vi "CSGaussmeter.setAuto.vi"(0 "i ref in":refnum<vi>, 7 "Auto":bool, 11 "error in (no error)":errorcluster) -> (4 "i ref out":refnum<vi>, 15 "error out":errorcluster)   [LabVIEW 2014, in "CSGaussmeter.lvlib"]
doc: "This VI sets the Auto Range ON or OFF. \n\nDurch das VI Auto_Range kann die automatische Messbereichswahl eingeschaltet werden."
uses:
  CSGaussmeter.lvlib
  CSCore/CSObj/CSObj.lvlib
  CSlibraries/UtilityLib/UtilityLib.lvlib
  CSinstr.lib/FH_55/FH 55.lvlib
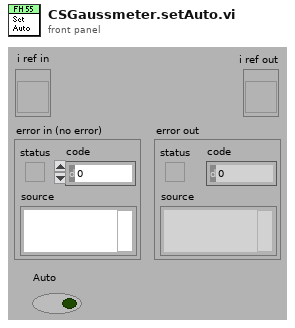
[diagram p1: front panel]
types:
  T1 = typedef "CSGaussmeter.lvlib/CSGaussmeter.i attribute.ctl" = cluster{"Name":string, "VISA Resource Name":refnum<visa-resource-name>, "actValues":cluster{" Limit":bool, "Unit ":T2, "Temp_Unit":T3, "Max":T4, " Filter":bool, " Peak":bool, " Auto_Range":bool, "Range":T5, " Rel":bool, " CTemp":bool, " CField":bool, "AC_DC ":bool, "Set_lower":cluster{"Numeric":dbl, "Cancel Button":bool, "Unit":T6}, "Set_upper":cluster{"Numeric":dbl, "Cancel Button":bool, "Unit":T6}, "Set_Rel":cluster{"Numeric":dbl, "Cancel Button":bool, "Unit":T6}, "Zero":bool, " Local":bool, "Reset":bool, " Init":bool}, "FH 55 Gauss-/Teslameter":T7, "MAX_Value":T8, "MIN_Value":T8, "Rel_Value":T8, "Array ":string[], "LIMU":dbl, " LIML":dbl, "Messwerte 2":string, "Messwerte ":cluster{"Numeric":i32, "OK Button":bool}, "serviceID":cluster{"Current ID":i32, "Unit ID":i32, "Temp ID":i32, "Name ID \n":i32, "Visa ID ":i32}, "setValues ":cluster{" Limit":bool, "Unit ":T2, "Temp_Unit":T3, "Max":T4, " Filter":bool, " Peak":bool, " Auto_Range":bool, "Range":T5, " Rel":bool, " CTemp":bool, " CField":bool, "AC_DC ":bool, "Set_lower":cluster{"Numeric":dbl, "Cancel Button":bool, "Unit":T6}, "Set_upper":cluster{"Numeric":dbl, "Cancel Button":bool, "Unit":T6}, "Set_Rel":cluster{"Numeric":dbl, "Cancel Button":bool, "Unit":T6}, "Zero":bool, " Local":bool, "Reset":bool, " Init":bool}}
  T2 = typedef "FH 55.lvlib/Unit.ctl" = enum16{"T", "G", "A/m"}
  T3 = typedef "FH 55.lvlib/Temp_Unit.ctl" = enum16{"Temp off", "Celsius", "Fahrenheit"}
  T4 = typedef "FH 55.lvlib/Max.ctl" = enum16{"MAX off", "Show MAX", "MAX/MIN"}
  T5 = typedef "FH 55.lvlib/Range.ctl" = enum16{"1", "2", "3", "4", "5", "6", "7"}
  T6 = typedef "FH 55.lvlib/Unit2.ctl" = enum16{"mT", "G", "kA/m"}
  T7 = typedef "FH 55.lvlib/Display.ctl" = cluster{"current value":string, "Limit":string, "Remote":string, "function ":string, "Cluster":cluster{"AC/DC":string, "Auto":string, "Filter":string, "Range":string, "Rel":string, "Peak":string}}
  T8 = typedef "FH 55.lvlib/Value_String.ctl" = cluster{"Numeric":dbl, "String":string}
  T9 = cluster{"VISA Resource Name":refnum<visa-resource-name>}
  T10 = typedef "FH 55.lvlib/VisaCluster.ctl" = cluster{"VISA Resource Name":refnum<visa-resource-name>}
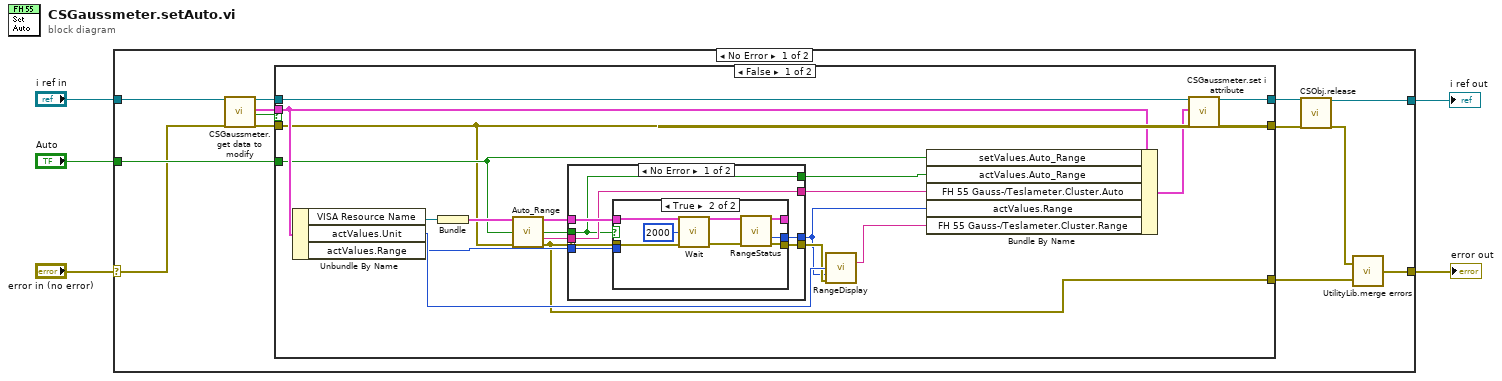
[diagram p0: block diagram]
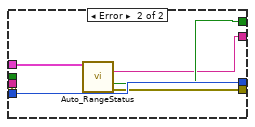
[diagram p3: hidden frame]
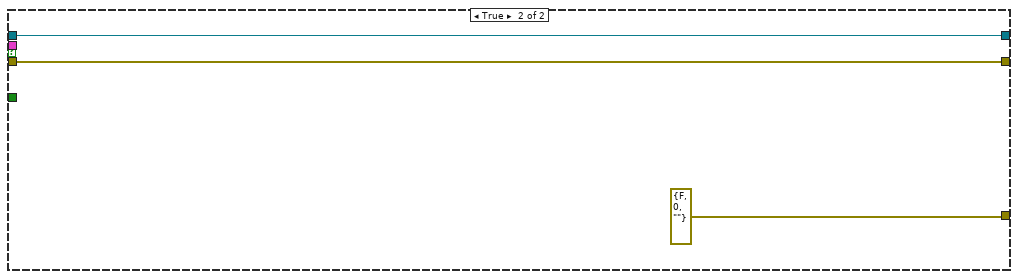
[diagram p4: hidden frame]
diagram:
  n1 = case shown="No Error" "error in (no error)" {
    selector: "error in (no error)" -> [w12 w64]
    tunnel: [w13 w64] -> w2
    tunnel: "i ref in" -> [w11 w65]
    tunnel: [w6 w65] -> w3
    tunnel: "Auto" -> [w15 _]
    frame No Error {
      n2 = call "CSGaussmeter.get data to modify.vi"("i ref in"=w11, "error in (no error)"=w12) -> ("i ref out"=w10:refnum<vi>, "i attribute"=w9:T1, "timed out"=w8:bool, "error out"=w7:errorcluster)  [unwired: 14 in]
      n3 = case shown="False" w8 {
        tunnel: w10 -> [w36 w62]
        tunnel: w7 -> [w28 w63]
        tunnel: w9 -> [w37 _]
        tunnel: [w27 w63] -> w16
        tunnel: [w34 w62] -> w18
        tunnel: w15 -> [w32 _]
        tunnel: [w20 errorcluster {"status"=FALSE, "code"=0, "source"=""} ("error out")] -> w14
        frame False {
          n4 = Unbundle By Name(w37) -> ("VISA Resource Name"=w38:refnum<visa-resource-name>, "actValues.Unit"=w30:T2, "actValues.Range"=w25:T5)
          n5 = Bundle("VISA Resource Name"=w38) -> (w33:T9)  [unwired: 1 in]
          n6 = call "Auto_Range.vi"("VisaCluster"=w33, "Auto_Range"=w32, "error in (no error)"=w28) -> ("VisaCluster"=w31:T10, "Auto"=w29:bool, "Display"=w24:string, "error out"=w20:errorcluster)  [unwired: 8 in, 1 out]
          n7 = case shown="No Error" w20 {
            selector: w20 -> [w43 _]
            tunnel: w31 -> [w45 w59]
            tunnel: w29 -> [w41 _]
            tunnel: w25 -> [w40 w60]
            tunnel: [w44 w60] -> w19
            tunnel: w24 -> [w42 _]
            tunnel: [w42 w57] -> w23
            tunnel: [w41 w58] -> w22
            tunnel: [w39 w56] -> w21
            frame No Error {
              n8 = case shown="True" w41 {
                tunnel: [w48 w49] -> w39
                tunnel: w43 -> [w48 w54]
                tunnel: w45 -> [w47 w53]
                tunnel: [w47 w52] -> _
                tunnel: [w46 w51] -> w44
                tunnel: w40 -> [w46 _]
                frame False {
                }
                frame True {
                  n9 = call "Wait.vi"("milliseconds to wait"=u32 2000, "error in (no error)"=w54) -> ("error out"=w50:errorcluster)  [unwired: 13 in]
                  n10 = call "RangeStatus.vi"("VisaCluster"=w53, "error in (no error)"=w50) -> ("VisaCluster"=w52:T10, "Range"=w51:T5, "error out"=w49:errorcluster)  [unwired: 10 in, 1 out]
                }
              }
            }
            frame Error {
              n11 = call "Auto_RangeStatus.vi"("VisaCluster"=w59) -> ("Display"=w57:string, "Auto_Range"=w58:bool, "error out"=w56:errorcluster)  [unwired: 10 in, 2 out]
            }
          }
          n12 = call "RangeDisplay.vi"("Unit"=w30, "Range"=w19, "error in (no error)"=w21) -> ("Display"=w26:string)  [unwired: 10 in, 2 out]
          n13 = Bundle By Name(cluster=w37, "setValues.Auto_Range"=w32, "actValues.Auto_Range"=w22, "FH 55 Gauss-/Teslameter.Cluster.Auto"=w23, "actValues.Range"=w19, "FH 55 Gauss-/Teslameter.Cluster.Range"=w26) -> (w35:T1)
          n14 = call "CSGaussmeter.set i attribute.vi"("i ref in"=w36, "i attribute"=w35, "error in (no error)"=w28) -> ("i ref out"=w34:refnum<vi>, "error out"=w27:errorcluster)  [unwired: 15 in]
        }
        frame True {
        }
      }
      n15 = call "CSObj.release.vi"("i ref in"=w18, "error in (no error)"=w16) -> ("i ref out"=w6:refnum<vi>, "error out"=w17:errorcluster)  [unwired: 16 in]
      n16 = call "UtilityLib.merge errors.vi"("error2 (no error)"=w14, "error1 (no error)"=w17) -> ("error out"=w13:errorcluster)
    }
    frame Error {
    }
  }
  "i ref out" <- w3
  "error out" <- w2
